vi "Merge Error.vi"(10 "Error":errorcluster, 11 "Base Queue in":refnum<class "Base Queue.lvclass">) -> (3 "Base Queue out":refnum<class "Base Queue.lvclass">)   [LabVIEW 2021, in "jettl.lvlib" / "Base Queue.lvlib" / "Base Queue.lvclass"]
uses:
  Base Queue.lvclass
  Base Queue.lvclass/Base Queue.ctl
  State/Error State/Error State.lvclass
  C:/git/jettl/jettl/jettl/Base Queue/State/Error State/Error State.lvclass
  C:/git/jettl/jettl/jettl/Base Queue/State/State/State.lvclass
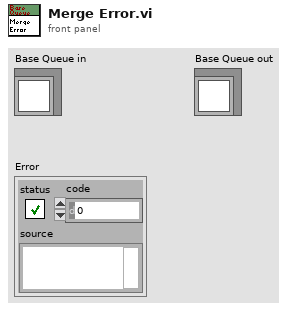
[diagram p1: front panel]
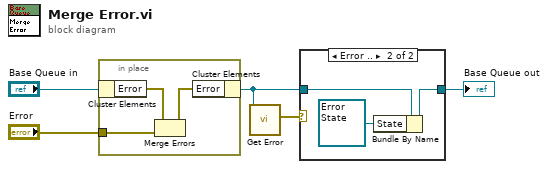
[diagram p0: block diagram]
diagram:
  n1 = in-place {
    in-place-border: "Error" -> [w6]
    n2 = in-place-cluster #1("Base Queue in") -> ("Error"=w8:errorcluster)
    n3 = Merge Errors(w8, w6) -> (w7:errorcluster)
    n4 = in-place-cluster #1("Error"=w7) -> (w2:refnum<class "Base Queue.lvclass">)
  }
  n5 = call-dynamic "Get Error.vi"("Base Queue in"=w2) -> ("Error"=w3:errorcluster)  [unwired: 10 in]
  n6 = case shown="Error .." w3 {
    tunnel: [w9 w11] -> w1
    tunnel: w2 -> [w9 w12]
    frame No Error {
    }
    frame Error {
      n7 = Bundle By Name(cluster=w12, "State"=refnum<class "Error State.lvclass"> refnum ("jettl.lvlib:jettl Queue Actor.lvlib:Error State.lvclass")) -> (w11:refnum<class "Base Queue.lvclass">)
    }
  }
  "Base Queue out" <- w1
